vi "Publish 0mq.vi"(8 "error in (no error)":errorcluster, 11 "ICS in":refnum<class "ICS.lvclass">) -> (0 "error out":errorcluster, 3 "ICS out":refnum<class "ICS.lvclass">)   [LabVIEW 2018, in "ICS.lvclass"]
uses:
  ICS.lvclass
  ICS.lvclass/ICS.ctl
  Message Queue/Message Cluster.ctl
  Messenger/Messenger.lvclass
  Motor/Motor.lvclass
  Message Queue/Message Queue.lvlib
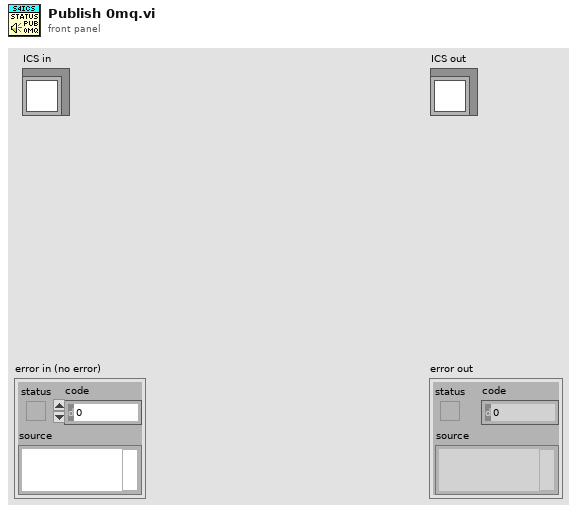
[diagram p1: front panel]
types:
  T1 = typedef "Message Queue.lvlib/Message Cluster.ctl" = cluster{"Message":string, "Message Data":variant}
  T2 = cluster{"mode":string, "condition":string, "position":string, "pos_name":string, "pos_id":string}
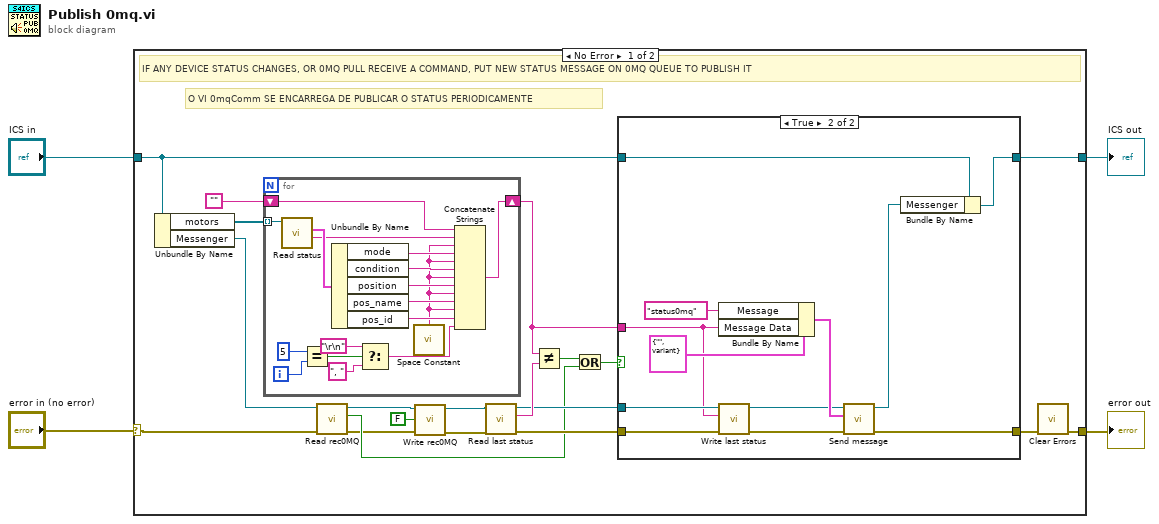
[diagram p0: block diagram]
diagram:
  n1 = case shown="No Error" "error in (no error)" {
    selector: "error in (no error)" -> [w11 w56]
    tunnel: [w16 w56] -> w3
    tunnel: [w17 w57] -> w1
    tunnel: "ICS in" -> [w18 w57]
    frame No Error {
      # "O VI 0mqComm SE ENCARREGA DE PUBLICAR O STATUS PERIODICAMENTE"
      # "IF ANY DEVICE STATUS CHANGES, OR 0MQ PULL RECEIVE A COMMAND, PUT NEW STATUS MESSAGE ON 0MQ QUEUE TO PUBLISH IT"
      n2 = Unbundle By Name(w18) -> ("motors"=w24:refnum<class "Motor.lvclass">[], "Messenger"=w12:refnum<class "Messenger.lvclass">)
      n3 = for {
        tunnel: w24 -> [w41] mode=indexing
        shift-right: [w26] -> w19
        shift-left: "" -> [w25]
        i -> [w28]
        n4 = call-dynamic "Read status.vi"("Motor in"=w41) -> ("name"=w39:string, "status"=w40:T2)  [unwired: 7 in, 2 out]
        n5 = Equal?(x=5, y=w28) -> (x = y?=w30:bool)
        n6 = Unbundle By Name(w40) -> ("mode"=w38:string, "condition"=w37:string, "position"=w36:string, "pos_name"=w35:string, "pos_id"=w34:string)
        n7 = Select(t="\r\n", s=w30, f=", ") -> (s? t:f=w27:string)
        n8 = call <vilib>:"Space Constant.vi"() -> ("String"=w33:string)
        n9 = Concatenate Strings(w25, w39, w33, w38, w33, w37, w33, w36, w33, w35, w33, w34, w27) -> (w26:string)
      }
      n10 = call-dynamic "Read rec0MQ.vi"("error in (no error)"=w11, "Messenger in"=w12) -> ("error out"=w7:errorcluster, "rec0MQ"=w10:bool, "Messenger out"=w9:refnum<class "Messenger.lvclass">)  [unwired: 7 in]
      n11 = call-dynamic "Write rec0MQ.vi"("error in (no error)"=w7, "rec0MQ"=FALSE, "Messenger in"=w9) -> ("error out"=w6:errorcluster, "Messenger out"=w8:refnum<class "Messenger.lvclass">)  [unwired: 7 in]
      n12 = call-dynamic "Read last status.vi"("error in (no error)"=w6, "Messenger in"=w8) -> ("error out"=w20:errorcluster, "last status"=w22:string, "Messenger out"=w21:refnum<class "Messenger.lvclass">)  [unwired: 7 in]
      n13 = Not Equal?(x=w19, y=w22) -> (x != y?=w14:bool)
      n14 = Or(x=w14, y=w10) -> (x .or. y?=w13:bool)
      n15 = case shown="True" w13 {
        tunnel: w21 -> [_ w51]
        tunnel: w20 -> [w43 w50]
        tunnel: w19 -> [_ w49]
        tunnel: [w43 w52] -> w15
        tunnel: w18 -> [w42 w46]
        tunnel: [w42 w45] -> w17
        frame False {
        }
        frame True {
          n16 = Bundle By Name(cluster=T1 {"Message"="", "Message Data"=variant} ("message"), "Message"="status0mq", "Message Data"=w49) -> (w53:T1)
          n17 = call-dynamic "Write last status.vi"("error in (no error)"=w50, "last status"=w49, "Messenger in"=w51) -> ("error out"=w47:errorcluster, "Messenger out"=w48:refnum<class "Messenger.lvclass">)  [unwired: 7 in]
          n18 = call-dynamic "Send message.vi"("error in (no error)"=w47, "message"=w53, "Messenger in"=w48) -> ("error out"=w52:errorcluster, "Messenger out"=w44:refnum<class "Messenger.lvclass">)  [unwired: 7 in]
          n19 = Bundle By Name(cluster=w46, "Messenger"=w44) -> (w45:refnum<class "ICS.lvclass">)
        }
      }
      n20 = call <vilib>:"Clear Errors.vi"("error in (no error)"=w15) -> ("error out"=w16:errorcluster)  [unwired: 5 in, 1 out]
    }
    frame Error {
    }
  }
  "error out" <- w3
  "ICS out" <- w1
